vi "PicoScope5000aExampleRapidBlockBulk-ajg.vi"() -> ()   [LabVIEW 2020]
panel:
  out "enabled array":i16[](array[numeric])
  out "wavefroms":waveform(dbl)[](graph)
  in  "Channel B Settings 2":T1={"Enabled"=TRUE, "Coupling"=1, "Range"=6, "Analogue Offset"=0.0} {"Range" items=["10 mV", "20 mV", "50 mV", "100 mV", "200 mV", "500 mV", "1 V", "2 V", "5 V", "10 V", "20 V", "50 V ", "100 V"]; "Coupling" items=["AC", "DC"]}
  in  "Rapid Block Acquisition Settings":T2={"preTriggerSamples"=0, "postTriggerSamples"=1000, "timebase"=2, "Down-Sample Mode"=0, "Down Sample Ratio"=1, "Number of Captures"=10} {"Down Sample Ratio" min=1 step=1; "Down-Sample Mode" items=["None"=0, "Aggregate"=1, "Decimate"=2, "Average"=4]}
  out "Device Info":T3
  out "Properties Panel":T4 {"Max Total Capture Time Available (sec)" format="%.3p"; "Sample Frequency" format="%.3p"; "Sample Rate" format="%.3p"; "Max Samples Available" format="%.3p"; "Total Capture Time (sec)" format="%.3p"}
  in  "Trigger Settings":T5={"Trigger Enabled"=FALSE, "Trigger Source"=enum."Channel A", "Trigger Threshold (volts)"=0.0, "Trigger Direction"=2, "Trigger Delay (samples)"=0, "Auto Trigger Time (ms)"=1000} {"Trigger Direction" items=["Rising"=2, "Falling"=3]}
  out "2-channel USB 3.0 device on non-USB 3.0 Port":bool=TRUE
  out "4-channel USB Powered":bool=TRUE
  in  "Serial Number":string
  in  "Use Serial Number":bool
  out "Number of Samples \nPer Capture":u32
  in  "Resolution":i32(ring)=1 items=["8-bit", "12-bit", "14-bit", "15-bit (max. 2 ch.)", "16-bit (max. 1 ch.)"]
  in  "Channel A Settings":T1={"Enabled"=TRUE, "Coupling"=1, "Range"=6, "Analogue Offset"=0.0} {"Range" items=["10 mV", "20 mV", "50 mV", "100 mV", "200 mV", "500 mV", "1 V", "2 V", "5 V", "10 V", "20 V", "50 V ", "100 V"]; "Coupling" items=["AC", "DC"]}
  out "Capture Complete":bool
  in  "stop":bool
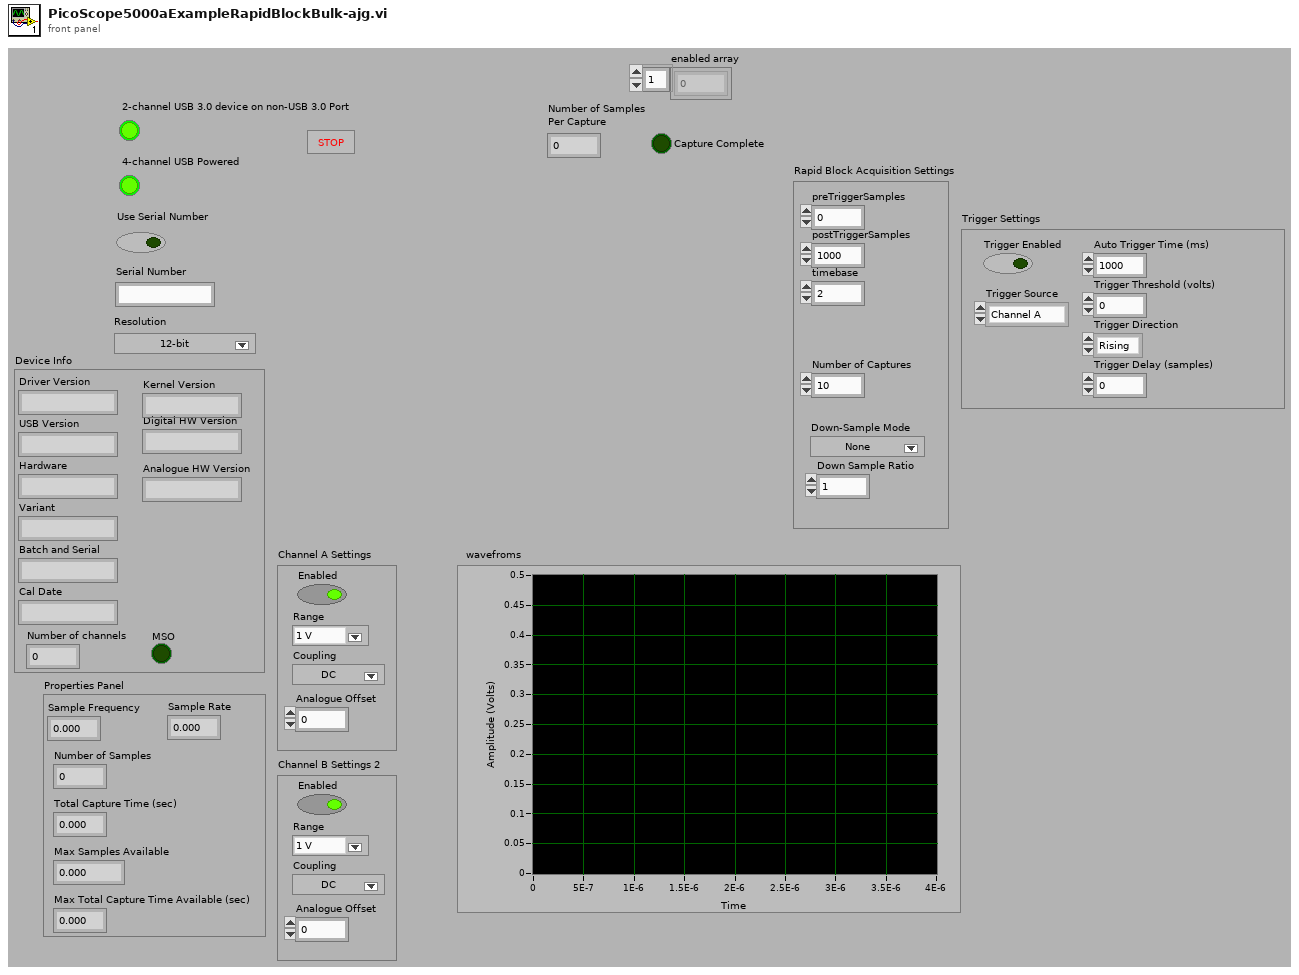
[diagram p1: front panel]
types:
  T1 = cluster{"Enabled":bool, "Coupling":i16, "Range":u16, "Analogue Offset":sgl}
  T2 = cluster{"preTriggerSamples":u32, "postTriggerSamples":u32, "timebase":u32, "Down-Sample Mode":i32, "Down Sample Ratio":u32, "Number of Captures":u32}
  T3 = cluster{"Driver Version":string, "USB Version":string, "Hardware":string, "Variant":string, "Batch and Serial":string, "Cal Date":string, "Kernel Version":string, "Digital HW Version":string, "Analogue HW Version":string, "MSO":bool, "Number of channels":i16}
  T4 = cluster{"Sample Frequency":sgl, "Sample Rate":sgl, "Max Samples Available":i32, "Number of Samples":u32, "Total Capture Time (sec) ":sgl, "Max Total Capture Time Available (sec)":sgl}
  T5 = cluster{"Trigger Enabled":bool, "Trigger Source":enum16{"Channel A", "Channel B", "Channel C", "Channel D", "Ext."}, "Trigger Threshold (volts)":dbl, "Trigger Direction":u16, "Trigger Delay (samples)":u32, "Auto Trigger Time (ms)":i16}
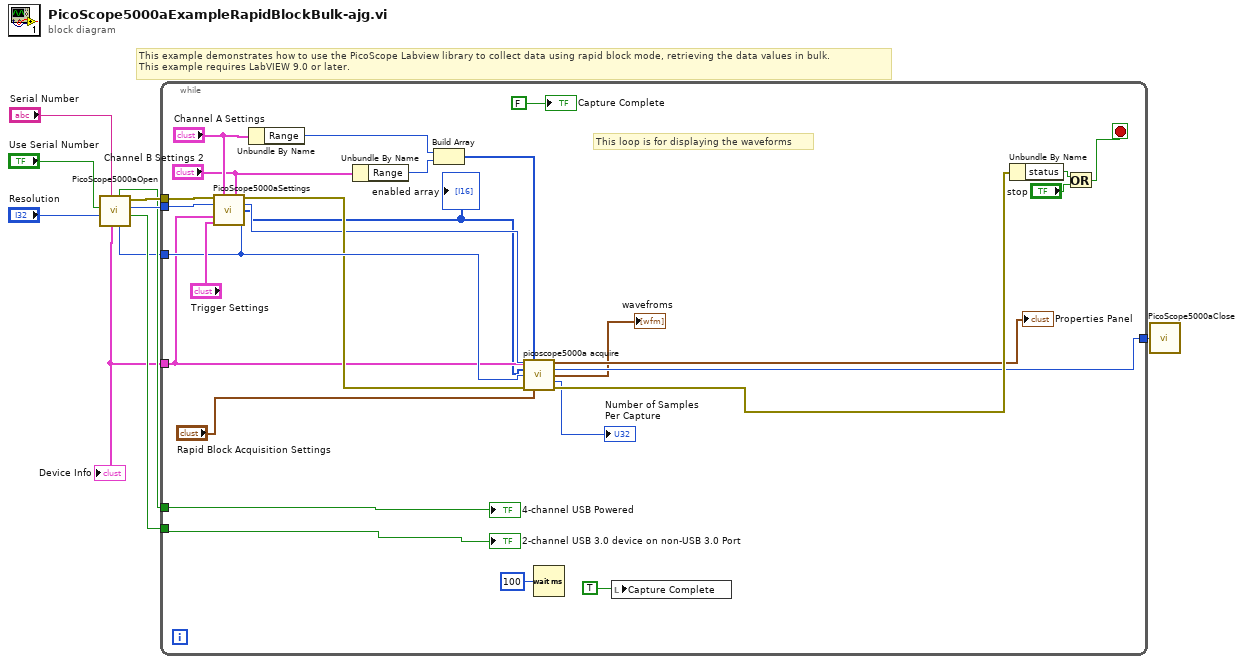
[diagram p0: block diagram]
diagram:
  # "This example demonstrates how to use the PicoScope Labview library to collect data using rapid block mode, retrieving the data values in bulk.\nThis example requires LabVIEW 9.0 or later."
  n1 = call "PicoScope5000aOpen.vi"("Serial Number"="Serial Number", "Resolution"="Resolution", "Use Serial Number"="Use Serial Number") -> ("USB Powered"=w7:bool, "handle"=w8:i16, "error out"=w9:errorcluster, "Max ADC value"=w2:i16, "USB 3.0 device on non-USB 3.0 Port"=w3:bool, "Device Info"=w1:T3)  [unwired: 3 in]
  "Device Info" <- w1
  n2 = while {
    tunnel: [w27] -> w10
    tunnel: w9 -> [w34]
    tunnel: w8 -> [w33]
    tunnel: w7 -> [w32]
    tunnel: w3 -> [w31]
    tunnel: w2 -> [w29]
    tunnel: w1 -> [w24]
    stop <- w37 stop-if-true
    # "This loop is for displaying the waveforms"
    n3 = call "PicoScope5000aSettings.vi"("error in"=w34, "Channel A Settings"="Channel A Settings", "Channel B Settings"="Channel B Settings 2", "handle in"=w33, "Device Info"=w24, "Trigger Settings"="Trigger Settings", "Max ADC value"=w29) -> ("error out"=w26:errorcluster, "handle out"=w25:i16, "enabled array"=w22:i16[])  [unwired: 6 in]
    "enabled array" <- w22
    n4 = Unbundle By Name("Channel A Settings") -> ("Range"=w13:u16)
    n5 = Unbundle By Name("Channel B Settings 2") -> ("Range"=w12:u16)
    n6 = Build Array(w13, w12) -> (w11:u16[])
    n7 = call "picoscope5000a acquire.vi"("handle in"=w25, "Ranges"=w11, "enabled array"=w22, "Max ADC value"=w29, "Device Info"=w24, "error in (no error)"=w26, "Rapid Block Acquisition Settings"="Rapid Block Acquisition Settings") -> ("Properties Panel"=→"Properties Panel":T4, "handle out 2"=w27:i16, "Waveform Data"=→"wavefroms":waveform(dbl)[], "Number of Samples \nPer Capture"=→"Number of Samples \nPer Capture":u32, "error out"=w35:errorcluster)  [unwired: 4 in]
    n8 = Wait (ms)(milliseconds to wait=u32 100) -> ()  [unwired: 1 out]
    n9 = local write "Capture Complete"(TRUE ("Capture Complete")) -> ()
    n10 = Unbundle By Name(w35) -> ("status"=w18:bool)
    n11 = Or(x=w18, y="stop") -> (x .or. y?=w37:bool)
    "Capture Complete" <- FALSE ("Capture Complete")
    "4-channel USB Powered" <- w31
    "2-channel USB 3.0 device on non-USB 3.0 Port" <- w32
  }
  n12 = call "PicoScope5000aClose.vi"("handle"=w10) -> ()
